vi "Velocity.vi"(10 "Timestep":dbl=0.1, 11 "Points In":dbl[][](array[numeric])) -> (3 "Velocity Out":dbl[][](array[numeric]))   [LabVIEW 2016]
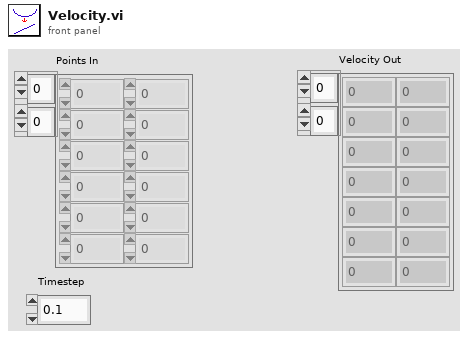
[diagram p1: front panel]
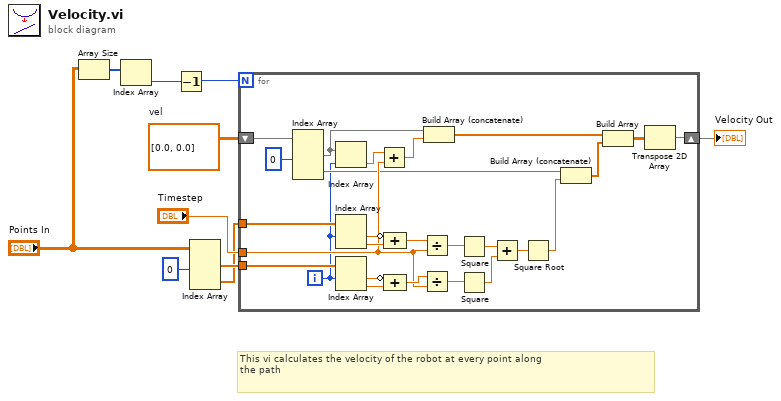
[diagram p0: block diagram]
diagram:
  w2 = dbl[][] [[0.0, 0.0]]  # vel
  # "This vi calculates the velocity of the robot at every point along\nthe path"
  n1 = Array Size(array="Points In") -> (size(s)=w10:i32[])
  n2 = Index Array(array=w10) -> (element=w9:i32)  [unwired: 1 in]
  n3 = Decrement(x=w9) -> (x-1=w8:i32)
  n4 = Index Array(array="Points In", index (col) #1=0 ("disabled index (col)")) -> (element #1=w5:dbl[], element #2=w4:dbl[])  [unwired: 3 in]
  n5 = for {
    N: w8 -> [_]
    tunnel: "Timestep" -> [w28]
    tunnel: w5 -> [w30]
    tunnel: w4 -> [w29]
    shift-right: [w12] -> w1
    shift-left: w2 -> [w16]
    i -> [w14]
    n6 = Index Array(array=w16, index (col) #1=0 ("disabled index (col)")) -> (element #1=w15:dbl[], element #2=w20:dbl[])  [unwired: 3 in]
    n7 = Index Array(array=w15, index=w14) -> (element=w13:dbl)
    n8 = Index Array(array=w29, index #1=w14) -> (element #1=w32:dbl, element #2=w33:dbl)  [unwired: 1 in]
    n9 = Index Array(array=w30, index #1=w14) -> (element #1=w35:dbl, element #2=w36:dbl)  [unwired: 1 in]
    n10 = Add(x=w13, y=w28) -> (x+y=w26:dbl)
    n11 = Compound Arithmetic op=ADD(invert w32, w33) -> (w31:dbl)
    n12 = Compound Arithmetic op=ADD(invert w35, w36) -> (w34:dbl)
    n13 = Divide(x=w31, y=w28) -> (x/y=w25:dbl)
    n14 = Divide(x=w34, y=w28) -> (x/y=w24:dbl)
    n15 = Build Array (concatenate)(w15, w26) -> (w19:dbl[])
    n16 = Square(x=w25) -> (x^2=w22:dbl)
    n17 = Square(x=w24) -> (x^2=w23:dbl)
    n18 = Add(x=w22, y=w23) -> (x+y=w21:dbl)
    n19 = Square Root(x=w21) -> (sqrt(x)=w17:dbl)
    n20 = Build Array (concatenate)(w20, w17) -> (w18:dbl[])
    n21 = Build Array(w19, w18) -> (w11:dbl[][])
    n22 = Transpose 2D Array(2D array=w11) -> (transposed array=w12:dbl[][])
  }
  "Velocity Out" <- w1
